vi "ReferenceSearch.vi"(0 "handle in":i32, 1 "UnitAddress(0)":u16, 2 "MotNr(0)":u8, 5 "error in":errorcluster) -> (14 "handle out":i32, 19 "error out":errorcluster)   [LabVIEW 2014, in "Sixpack - Driver.lvlib"]
doc: "Der Motor fährt in der vorkonfigurierten Richtung mit der Geschwindigkeit VMin, bis der Referenzpunkt über den Referenzpunktschalter eindeutig identifiziert wurde. Die Position wird dann auf null gesetzt. Wenn das Flag STOPAFTERREF = 0 (siehe SetRefSearchParameters), fährt der Motor nach Ende der Referenzfahrt wieder an die Position, von der er die Referenzfahrt gestartet hat."
uses:
  Sixpack - Driver.lvlib
  DLL/PackDLL.dll
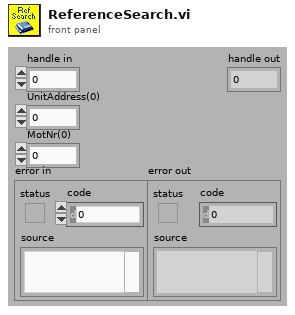
[diagram p1: front panel]
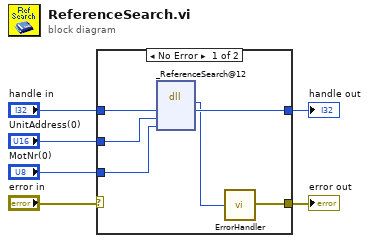
[diagram p0: block diagram]
diagram:
  n1 = case shown="No Error" "error in" {
    selector: "error in" -> [_ w13]
    tunnel: "handle in" -> [w12 w14]
    tunnel: [w11 w14] -> w5
    tunnel: "UnitAddress(0)" -> [w10 _]
    tunnel: "MotNr(0)" -> [w9 _]
    tunnel: [w7 w13] -> w2
    frame No Error {
      n2 = dll-call lib="D:/CS-Source/LV2014/GPL/instr.lib/SixPack/PackDLL/DLL/PackDLL.dll" fn="_ReferenceSearch@12" label="ReferenceSearch"("HANDLE"=w12, "UnitAddress"=w10, "MotNr"=w9) -> ("BOOLEAN"=w8:i8, "HANDLE"=w11:i32)  [unwired: 5 in, 2 out]
      n3 = call "ErrorHandler.vi"("BOOLEAN"=w8) -> ("error out"=w7:errorcluster)
    }
    frame Error {
    }
  }
  "handle out" <- w5
  "error out" <- w2
